vi "Contains Object Entry.vi"(8 "error in":errorcluster, 10 "OD Index":u16 format="%.0x", 11 "Obj Dict in":refnum<class "Object Dictionary.lvclass">) -> (0 "error out":errorcluster, 2 "Contains":bool, 3 "Obj Dict out":refnum<class "Object Dictionary.lvclass">)   [LabVIEW 2020, in "CANopen.lvlib" / "Object Dictionary.lvclass"]
uses:
  Object Dictionary.lvclass
  Object Dictionary.lvclass/Object Dictionary.ctl
  Ordered-Dictionary/Ordered Object Dictionary/Source/Ordered Object Dictionary.lvclass
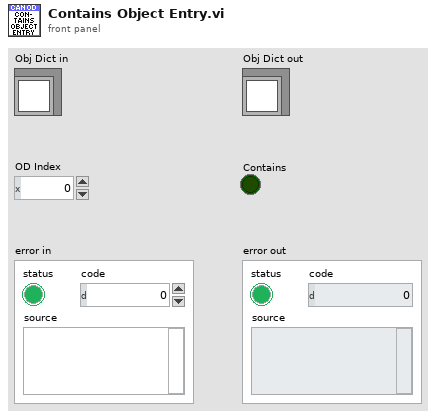
[diagram p1: front panel]
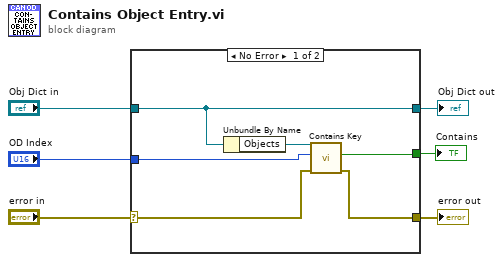
[diagram p0: block diagram]
diagram:
  n1 = case shown="No Error" "error in" {
    selector: "error in" -> [w10 w14]
    tunnel: [w9 w14] -> w3
    tunnel: [w12 w13] -> w5
    tunnel: "Obj Dict in" -> [w12 w13]
    tunnel: [w8 _] -> w2
    tunnel: "OD Index" -> [w7 _]
    frame No Error {
      n2 = Unbundle By Name(w12) -> ("Objects"=w11:refnum<class "Ordered Object Dictionary.lvclass">)
      n3 = call "Contains Key.vi"("error in"=w10, "Key"=w7, "Ordered Object Dictionary in"=w11) -> ("error out"=w9:errorcluster, "Contains"=w8:bool)  [unwired: 6 in, 1 out]
    }
    frame Error {
    }
  }
  "Obj Dict out" <- w5
  "error out" <- w3
  "Contains" <- w2
